vi "GUI - Start Test (SubVI).vi"(7 "References":T1) -> ()   [LabVIEW 2010]
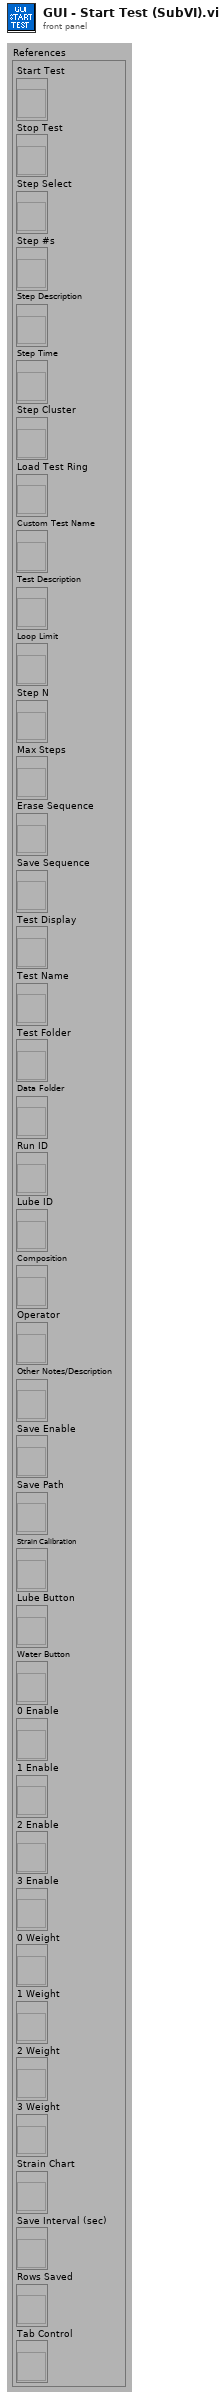
[diagram p1: front panel]
types:
  T1 = cluster{"Start Test":refnum<vi>, "Stop Test":refnum<vi>, "Step Select":refnum<vi>, "Step #s":refnum<vi>, "Step Description":refnum<vi>, "Step Time":refnum<vi>, "Step Cluster":refnum<vi>, "Load Test Ring":refnum<vi>, "Custom Test Name":refnum<vi>, "Test Description":refnum<vi>, "Loop Limit":refnum<vi>, "Step N":refnum<vi>, "Max Steps":refnum<vi>, "Erase Sequence":refnum<vi>, "Save Sequence":refnum<vi>, "Test Display":refnum<vi>, "Test Name":refnum<vi>, "Test Folder":refnum<vi>, "Data Folder":refnum<vi>, "Run ID":refnum<vi>, "Lube ID":refnum<vi>, "Composition":refnum<vi>, "Operator":refnum<vi>, "Other Notes/Description":refnum<vi>, "Save Enable":refnum<vi>, "Save Path":refnum<vi>, "Strain Calibration":refnum<vi>, "Lube Button":refnum<vi>, "Water Button":refnum<vi>, "0 Enable":refnum<vi>, "1 Enable":refnum<vi>, "2 Enable":refnum<vi>, "3 Enable":refnum<vi>, "0 Weight":refnum<vi>, "1 Weight":refnum<vi>, "2 Weight":refnum<vi>, "3 Weight":refnum<vi>, "Strain Chart":refnum<vi>, "Save Interval (sec)":refnum<vi>, "Rows Saved":refnum<vi>, "Tab Control":refnum<vi>}
  T2 = enum8{"Enabled", "Disabled", "Disabled and Grayed Out"}
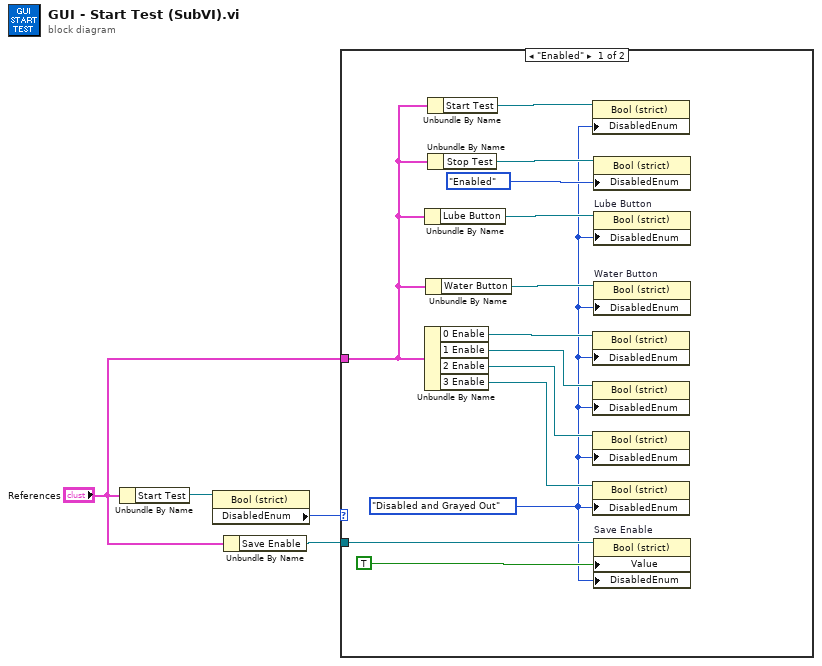
[diagram p0: block diagram]
diagram:
  n1 = Unbundle By Name("References") -> ("Start Test"=w4:refnum<vi>)
  n2 = property class="Bool (strict)"(reference=w4) -> ("DisabledEnum"=w2:T2)  [unwired: 1 in, 2 out]
  n3 = Unbundle By Name("References") -> ("Save Enable"=w3:refnum<vi>)
  n4 = case shown="\"Enabled\"" w2 {
    tunnel: w3 -> [w16 _]
    tunnel: "References" -> [w6 _]
    frame "Enabled" {
      w5 = T2."Disabled and Grayed Out" ("Disabled")
      n5 = Unbundle By Name(w6) -> ("Lube Button"=w11:refnum<vi>)
      n6 = Unbundle By Name(w6) -> ("0 Enable"=w15:refnum<vi>, "1 Enable"=w14:refnum<vi>, "2 Enable"=w13:refnum<vi>, "3 Enable"=w12:refnum<vi>)
      n7 = Unbundle By Name(w6) -> ("Water Button"=w10:refnum<vi>)
      n8 = Unbundle By Name(w6) -> ("Start Test"=w9:refnum<vi>)
      n9 = Unbundle By Name(w6) -> ("Stop Test"=w8:refnum<vi>)
      n10 = property class="Bool (strict)"(reference=w9, "DisabledEnum"=w5) -> ()  [unwired: 1 in, 2 out]
      n11 = property class="Bool (strict)"(reference=w15, "DisabledEnum"=w5) -> ()  [unwired: 1 in, 2 out]
      n12 = property class="Bool (strict)"(reference=w14, "DisabledEnum"=w5) -> ()  [unwired: 1 in, 2 out]
      n13 = property class="Bool (strict)"(reference=w13, "DisabledEnum"=w5) -> ()  [unwired: 1 in, 2 out]
      n14 = property class="Bool (strict)"(reference=w12, "DisabledEnum"=w5) -> ()  [unwired: 1 in, 2 out]
      n15 = property class="Bool (strict)"(reference=w8, "DisabledEnum"=T2."Enabled") -> ()  [unwired: 1 in, 2 out]
      n16 = property on="Lube Button" class="Bool (strict)"(reference=w11, "DisabledEnum"=w5) -> ()  [unwired: 1 in, 2 out]
      n17 = property on="Water Button" class="Bool (strict)"(reference=w10, "DisabledEnum"=w5) -> ()  [unwired: 1 in, 2 out]
      n18 = property on="Save Enable" class="Bool (strict)"(reference=w16, "Value"=TRUE, "DisabledEnum"=w5) -> ()  [unwired: 1 in, 2 out]
    }
    frame "Disabled", Default {
    }
  }
